vi "AlliGator Get Image Destination File Path.vi"(6 "Image File Extension":string, 7 "Image Name Prefix":string, 8 "Error In":errorcluster, 9 "Current Data Set":i32, 10 "Time-Series Paths":path[](array[path]), 11 "Single Data Point Path":path) -> (0 "Error Out":errorcluster, 3 "Image File Path":path)   [LabVIEW 2021, in "AlliGator Source Image.lvlib"]
doc: "Builds path to save a front panel object's image based on its source and the current dataset."
uses:
  AlliGator Source Image.lvlib
  AlliGator Files.lvlib
panel:
  # "see the AlliGator License on the block diagram (Ctrl+E or Window:Show Block Diagram)"
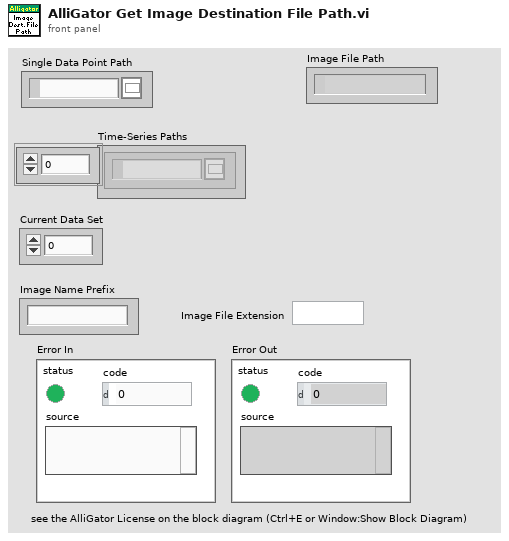
[diagram p1: front panel]
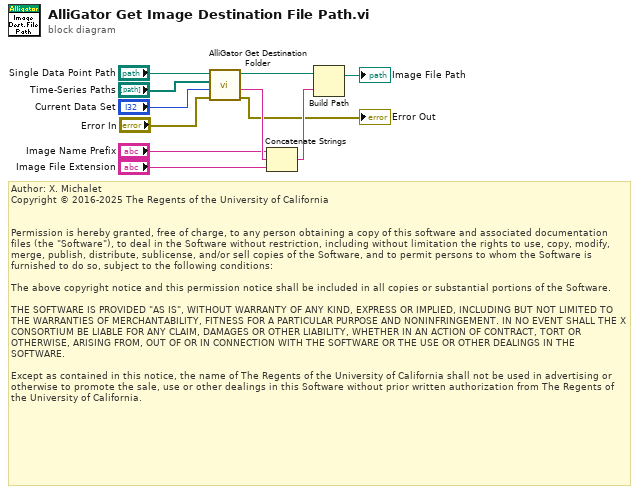
[diagram p0: block diagram]
diagram:
  # "Author: X. Michalet\nCopyright © 2016-2025 The Regents of the University of California\n \n\nPermission is hereby granted, free of charge, to any person obtaining a copy of this software and associated documentation files (the \"Software\"), to deal in the Software without restriction, including without limitation the rights to use, copy, modify, merge, publish, distribute, sublicense, and/or sell copies of the Software, and to permit persons to whom the Software is furnished to do so, subject to the following conditions:\n\nThe above copyright notice and this permission notice shall be included in all copies or substantial portions of the Software.\n\nTHE SOFTWARE IS PROVIDED \"AS IS\", WITHOUT WARRANTY OF ANY KIND, EXPRESS OR IMPLIED, INCLUDING BUT NOT LIMITED TO THE WARRANTIES OF MERCHANTABILITY, FITNESS FOR A PARTICULAR PURPOSE AND NONINFRINGEMENT. IN NO EVENT SHALL THE X CONSORTIUM BE LIABLE FOR ANY CLAIM, DAMAGES OR OTHER LIABILITY, WHETHER IN AN ACTION OF CONTRACT, TORT OR OTHERWISE, ARISING FROM, OUT OF OR IN CONNECTION WITH THE SOFTWARE OR THE USE OR OTHER DEALINGS IN THE SOFTWARE.\n\nExcept as contained in this notice, the name of The Regents of the University of California shall not be used in advertising or otherwise to promote the sale, use or other dealings in this Software without prior written authorization from The Regents of the University of California."
  n1 = call "AlliGator Get Destination Folder.vi"("Error In"="Error In", "Current Data Set (-1: single)"="Current Data Set", "Time-Series Paths"="Time-Series Paths", "Single Data Point Path"="Single Data Point Path") -> ("Error Out"=→"Error Out":errorcluster, "Data Point Name"=w11:string, "Destination Folder path"=w4:path)  [unwired: 5 in]
  n2 = Concatenate Strings("Image Name Prefix", w11, "Image File Extension") -> (w5:string)
  n3 = Build Path(base path=w4, name or relative path=w5) -> (appended path=→"Image File Path":path)
